vi "Check SBR.vi"(8 "error in (no error)":errorcluster {"code" format="%.0x"}, 11 "VISA session":refnum<visa-resource-name>) -> (0 "error out":errorcluster {"code" format="%.0x"}, 1 "Read SBR":T1, 3 "dup VISA session":refnum<visa-resource-name>)   [LabVIEW 2011]
doc: "Checks the instrument's IEEE-488.2 Status-Byte Register. The Status Byte Register indicator enables the associated events.\n\nThe bits in the event register are cleared automatically after calling this VI.\n\nNotes: \n(1) You can call this VI between a VISA Write sending a query command and the corresponding VISA Read without causing a query error on your instrument.\n(2) Calling this VI does NOT clear the contents of the status byte register. Sending *CLS will clear all the registers."
uses:
  Low Level/Status Byte Indicator.ctl
panel:
  # "Status Byte Register (SBR)"
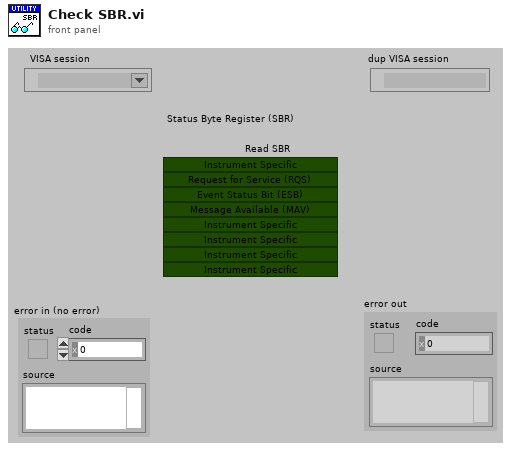
[diagram p1: front panel]
types:
  T1 = typedef "Status Byte Indicator.ctl" = cluster{"Instrument Specific (1)":bool, "Instrument Specific (2)":bool, "Instrument Specific (4)":bool, "Instrument Specific (8)":bool, "Message Available (16)":bool, "Event Status Bit (32)":bool, "Request for Service (32)":bool, "Instrument Specific (128)":bool}
  T2 = cluster{"[0]":bool, "[1]":bool, "[2]":bool, "[3]":bool, "[4]":bool, "[5]":bool, "[6]":bool, "[7]":bool}
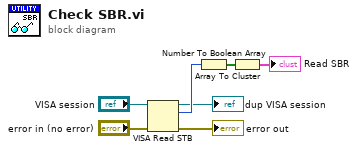
[diagram p0: block diagram]
diagram:
  n1 = VISA Read STB(8:"error in (no error)", 11:"VISA session") -> (0:→"error out":errorcluster, 2:w5:u16, 3:→"dup VISA session":refnum<visa-resource-name>)
  n2 = Number To Boolean Array(number=w5) -> (Boolean array=w7:bool[])
  n3 = Array To Cluster(array=w7) -> (cluster=→"Read SBR":T2)
